vi "Multi-device Synchronous AI and AO.vi"() -> ()   [LabVIEW 2009]
uses:
  <vilib>/DAQmx/write.llb/DAQmx Write (Analog Wfm 1Chan NSamp).vi
  <vilib>/DAQmx/configure/timing.llb/DAQmx Timing (Sample Clock).vi
  <vilib>/DAQmx/create/channels.llb/DAQmx Create Channel (AO-Voltage-Basic).vi
  <vilib>/DAQmx/create/channels.llb/DAQmx Create Channel (AI-Temperature-Thermocouple).vi
  <vilib>/DAQmx/read.llb/DAQmx Read (Analog 1D DBL 1Chan NSamp).vi
  Program Files/National Instruments/LabVIEW 2009/resource/objmgr/daqmx.rc
  <vilib>/measure/NI_MABase.lvlib
panel:
  out "data":dbl[](graph)
  out "signal out":waveform(dbl)(graph)
  in  "stop":bool
  in  "output rate":dbl(slide)=50.0 scale=10.0..50.0
  in  "AI channel":tag="cDAQ1Mod1/ai1"
  in  "AO channel":tag="Dev1/ao0"
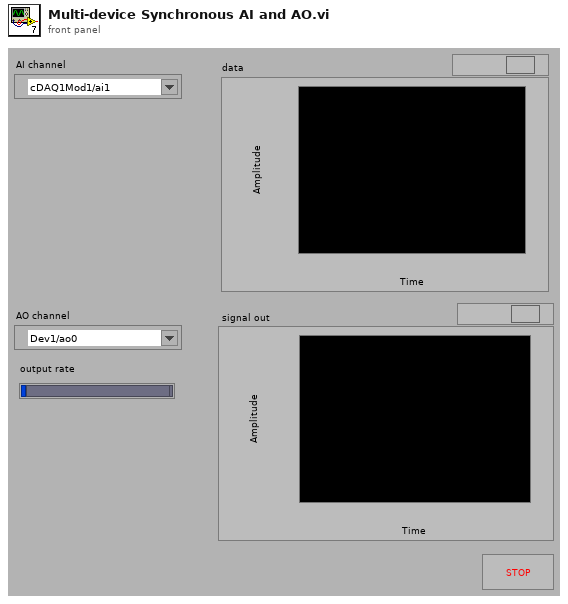
[diagram p1: front panel]
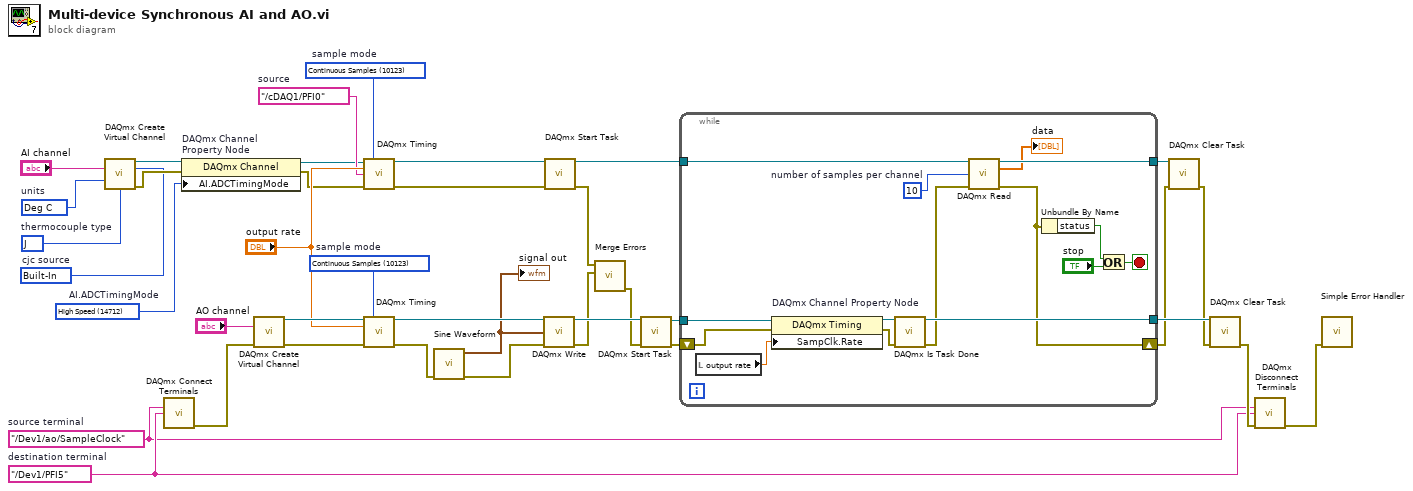
[diagram p0: block diagram]
diagram:
  w1 = 10143 items=["Deg C"=10143, "Deg F"=10144, "Kelvins"=10325, "Deg R"=10145, "From Custom Scale"=10065]  # units
  w2 = 10200 items=["Built-In"=10200, "Constant Value"=10116, "Channel"=10113]  # cjc source
  w3 = 10072 items=["J"=10072, "K"=10073, "N"=10077, "R"=10082, "S"=10085, "T"=10086, "B"=10047, "E"=10055]  # thermocouple type
  w4 = 14712 items=["High Resolution"=10195, "High Speed"=14712, "Best 50 Hz Rejection"=14713, "Best 60 Hz Rejection"=14714]  # AI.ADCTimingMode
  w11 = tag "/Dev1/PFI5"  # destination terminal
  w10 = tag "/Dev1/ao/SampleClock"  # source terminal
  w14 = tag "/cDAQ1/PFI0"  # source
  w23 = 10123 items=["Finite Samples"=10178, "Continuous Samples"=10123, "Hardware Timed Single Point"=12522]  # sample mode
  w24 = 10123 items=["Finite Samples"=10178, "Continuous Samples"=10123, "Hardware Timed Single Point"=12522]  # sample mode
  n1 = call-poly <vilib>:"DAQmx Create Virtual Channel.vi"("physical channels"="AI channel", "cjc source"=w2, "units"=w1, "thermocouple type"=w3) -> ("task out"=w8:refnum<k21>, "error out"=w6:errorcluster)  [unwired: 10 in]
  n2 = call <vilib>:"DAQmx Connect Terminals.vi"("source terminal"=w10, "destination terminal"=w11) -> ("error out"=w13:errorcluster)  [unwired: 13 in]
  n3 = property on="DAQmx Channel\nProperty Node" class="DAQmx Channel"(reference=w8, error in=w6, "AI.ADCTimingMode"=w4) -> (reference out=w7:refnum<k21>, error out=w5:errorcluster)
  n4 = call-poly <vilib>:"DAQmx Create Virtual Channel.vi"("physical channels"="AO channel", "error in"=w13) -> ("task out"=w17:refnum<k21>, "error out"=w16:errorcluster)  [unwired: 12 in]
  n5 = call-poly <vilib>:"DAQmx Timing.vi"("task/channels in"=w7, "sample mode"=w24, "rate"="output rate", "source"=w14, "error in"=w5) -> ("task out"=w31:refnum<k21>, "error out"=w18:errorcluster)  [unwired: 9 in]
  n6 = call-poly <vilib>:"DAQmx Timing.vi"("task/channels in"=w17, "sample mode"=w23, "rate"="output rate", "error in"=w16) -> ("task out"=w30:refnum<k21>, "error out"=w27:errorcluster)  [unwired: 10 in]
  n7 = call <vilib>:"Sine Waveform.vi"("error in (no error)"=w27) -> ("error out"=w26:errorcluster, "signal out"=w25:waveform(dbl))  [unwired: 9 in]
  "signal out" <- w25
  n8 = call-poly <vilib>:"DAQmx Write.vi"("task/channels in"=w30, "data"=w25, "error in"=w26) -> ("task out"=w36:refnum<k21>, "error out"=w20:errorcluster)  [unwired: 10 in, 1 out]
  n9 = call <vilib>:"DAQmx Start Task.vi"("task/channels in"=w31, "error in"=w18) -> ("task out"=w35:refnum<k21>, "error out"=w19:errorcluster)  [unwired: 12 in]
  n10 = call <vilib>:"Merge Errors.vi"("error in 2 (no error)"=w20, "error in 1 (no error)"=w19) -> ("error out"=w21:errorcluster)  [unwired: 5 in]
  n11 = call <vilib>:"DAQmx Start Task.vi"("task/channels in"=w36, "error in"=w21) -> ("task out"=w37:refnum<k21>, "error out"=w22:errorcluster)  [unwired: 12 in]
  n12 = while {
    tunnel: [w52] -> w38
    tunnel: w37 -> [w50]
    tunnel: w35 -> [w49]
    tunnel: [w48] -> w34
    shift-right: [w46] -> w29
    shift-left: w22 -> [w40]
    stop <- w43 stop-if-true
    w41 = 10  # number of samples per channel
    n13 = local read "output rate"() -> (w42:dbl)
    n14 = property on="DAQmx Channel Property Node" class="DAQmx Timing"(reference=w50, error in=w40, "SampClk.Rate"=w42) -> (reference out=w51:refnum<k21>, error out=w53:errorcluster)
    n15 = call <vilib>:"DAQmx Is Task Done.vi"("task/channels in"=w51, "error in"=w53) -> ("task out"=w52:refnum<k21>, "error out"=w47:errorcluster)  [unwired: 11 in, 1 out]
    n16 = call-poly <vilib>:"DAQmx Read.vi"("task/channels in"=w49, "number of samples per channel"=w41, "error in"=w47) -> ("task out"=w48:refnum<k21>, "data"=→"data":dbl[], "error out"=w46:errorcluster)  [unwired: 10 in]
    n17 = Unbundle By Name "Unbundle By Name"(w46) -> ("status"=w45:bool)
    n18 = Or(x=w45, y="stop") -> (x .or. y?=w43:bool)
  }
  n19 = call <vilib>:"DAQmx Clear Task.vi"("task in"=w34, "error in"=w29) -> ("error out"=w28:errorcluster)  [unwired: 13 in]
  n20 = call <vilib>:"DAQmx Clear Task.vi"("task in"=w38, "error in"=w28) -> ("error out"=w12:errorcluster)  [unwired: 13 in]
  n21 = call <vilib>:"DAQmx Disconnect Terminals.vi"("source terminal"=w10, "destination terminal"=w11, "error in"=w12) -> ("error out"=w9:errorcluster)  [unwired: 12 in]
  n22 = call <vilib>:"Simple Error Handler.vi"("error in (no error)"=w9) -> ()  [unwired: 4 in, 5 out]
